vi "GetPeak.vi"(8 "error in (no error)":errorcluster, 11 "Instruments in":refnum<class "Instruments.lvclass">) -> (0 "error out":errorcluster, 2 "Peak Wl":dbl, 3 "Instruments out":refnum<class "Instruments.lvclass">)   [LabVIEW 2012, in "Instruments.lvclass"]
uses:
  Instruments.lvclass
  Instruments.lvclass/Instruments.ctl
panel:
  out "max value":dbl
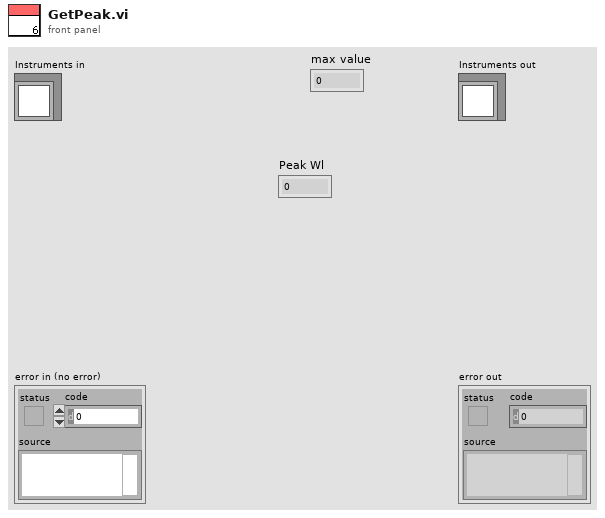
[diagram p1: front panel]
types:
  T1 = typedef "USB4000_Data.ctl" = cluster{"Wrapper Out":u32, "Number of Spectrometers":i32, "Wavelength":dbl[], "EL Spectrum":dbl[], "Int Time (usec)":i32, bool, "Background":dbl[]}
  T2 = typedef "Config.ctl" = cluster{"IntTime":i32, "Samples":i32, "PowerMin":dbl, "KneeMin":dbl, "KneeMax":dbl}
  T3 = cluster{"Keithley_Param":cluster{"Start Current,mA":dbl, "Stop Current,mA":dbl, "Voltage Compliance,V":dbl, "GPIB":string}, "USB4000_Param":cluster{"Integration Time":i32, "Wl min,nm":dbl, "Wl max,nm":dbl, "USB4000":T1}, "Ophir_Param":cluster{"VISA resource name":refnum<visa-resource-name>, "Calibration Wl":dbl}, "Config":T2}
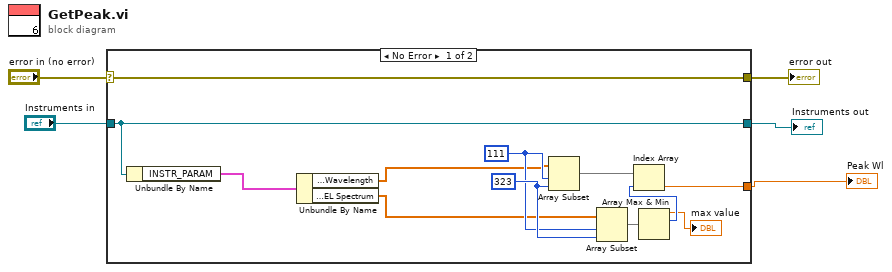
[diagram p0: block diagram]
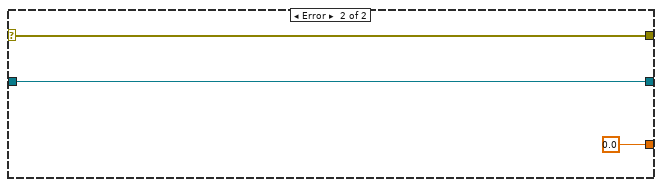
[diagram p2: hidden frame]
diagram:
  n1 = case shown="No Error" "error in (no error)" {
    selector: "error in (no error)" -> [w17 w20]
    tunnel: [w17 w20] -> w4
    tunnel: [w13 w19] -> w2
    tunnel: "Instruments in" -> [w13 w19]
    tunnel: [w12 0.0] -> w1
    frame No Error {
      w9 = 111 ("index")
      w10 = 323 ("length")
      n2 = Unbundle By Name(w13) -> ("INSTR_PARAM"=w6:T3)
      n3 = Unbundle By Name(w6) -> ("USB4000_Param.USB4000.Wavelength"=w8:dbl[], "USB4000_Param.USB4000.EL Spectrum"=w7:dbl[])
      n4 = Array Subset(array=w8, index=w9, length=w10) -> (w15:dbl[])
      n5 = Array Subset(array=w7, index=w9, length=w10) -> (w16:dbl[])
      n6 = Array Max & Min(array=w16) -> (max value=→"max value":dbl, max index (indices)=w14:i32)  [unwired: 2 out]
      n7 = Index Array(array=w15, index=w14) -> (element=w12:dbl)
    }
    frame Error {
    }
  }
  "error out" <- w4
  "Instruments out" <- w2
  "Peak Wl" <- w1
